vi "数组合并.vi"() -> ()   [LabVIEW 2023]
panel:
  in  "Numeric 2":dbl
  out "output array 4":dbl[](array[numeric])
  in  "Array 6":dbl[](array[numeric])
  in  "Numeric":dbl
  out "output array 3":dbl[](array[numeric])
  in  "Array 5":dbl[](array[numeric])
  out "appended array":dbl[][](array[numeric])
  out "output array 2":dbl[](array[numeric])
  in  "Array 4":dbl[](array[numeric])
  in  "Array 3":dbl[](array[numeric])
  in  "Array 2":dbl[](array[numeric])
  in  "Array":dbl[](array[numeric])
  # "数组合并"
  # "数字数组合并"
  # "Build Array"
  # "数字数组合并"
  # "Insert array"
  # "数字数组合并"
  # "build array"
  # "数字数组合并"
  # "insert  array"
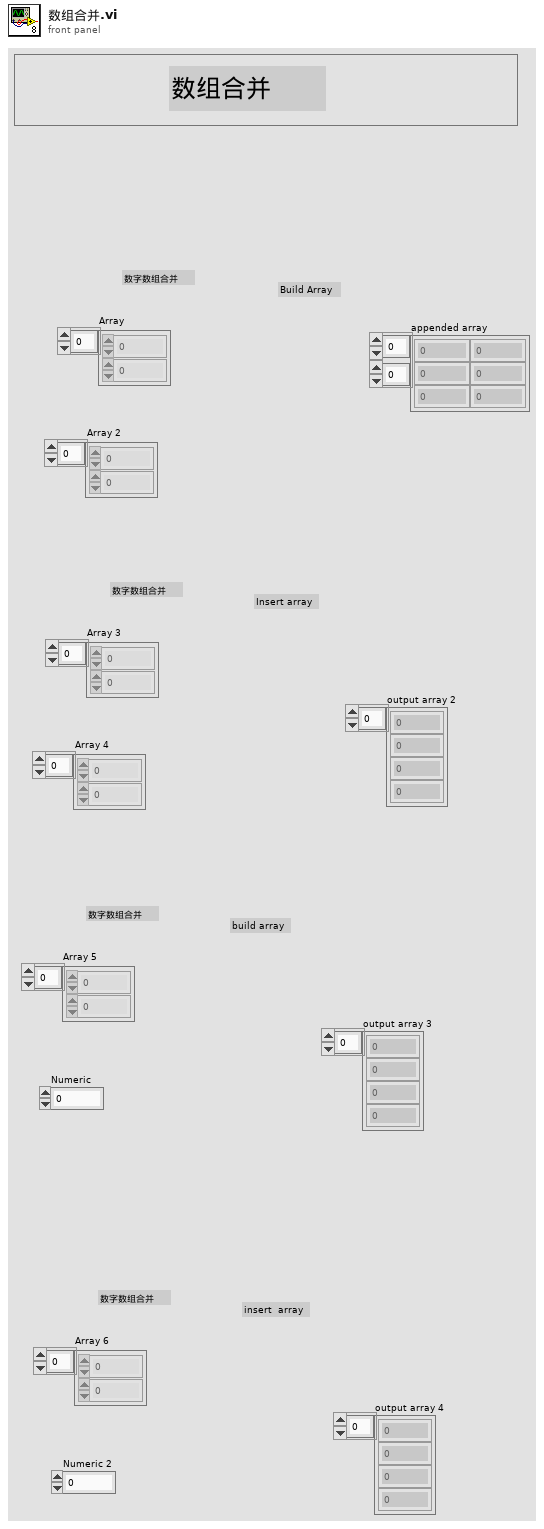
[diagram p1: front panel]
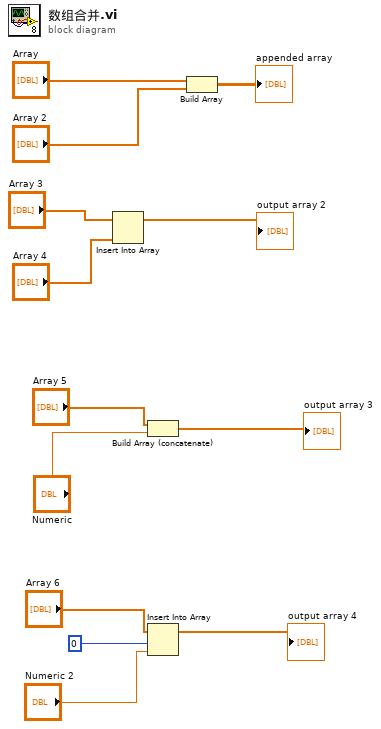
[diagram p0: block diagram]
diagram:
  n1 = Insert Into Array(array="Array 3", new element="Array 4") -> (→"output array 2":dbl[])  [unwired: 1 in]
  n2 = Build Array (concatenate)("Array 5", "Numeric") -> (→"output array 3":dbl[])
  n3 = Insert Into Array(array="Array 6", index=0, new element="Numeric 2") -> (→"output array 4":dbl[])
  n4 = Build Array("Array", "Array 2") -> (→"appended array":dbl[][])
